vi "Main Monitor Loop.vi"(5 "tdms file out":refnum<k34>, 7 "Message Queue":refnum<queue>, 8 "error in (no error)":errorcluster, 10 "DATA ARRAY":dbl[][](array[numeric]), 11 "main ref":T1) -> (0 "error out":errorcluster, 2 "DATA ARRAY OUT":dbl[][](array[numeric]))   [LabVIEW 2025]
uses:
  v06/controls/LAB-IQ UI Data.ctl
  Traction Loop/Traction Receipe Enum.ctl
  support/Message Queue/Message Cluster.ctl
  Temperature/Temperature enum.ctl
  <vilib>/Utility/error.llb/Trim Whitespace One-Sided.vi
  support/Message Queue/Enqueue Message (Single).vi
  support/Message Queue/LAB-IQ Message Queue.lvlib
panel:
  out "error out 4":errorcluster
  out "ELAPSED INDICATION":bool
  out "error out 3":errorcluster
  out "output array":dbl[][](array[numeric])
  out "error out 2":errorcluster
  in  "Checkbox":bool
  out "Time elapsed":bool
  out "Test Stop Temp":bool
  out "DepthZ":dbl
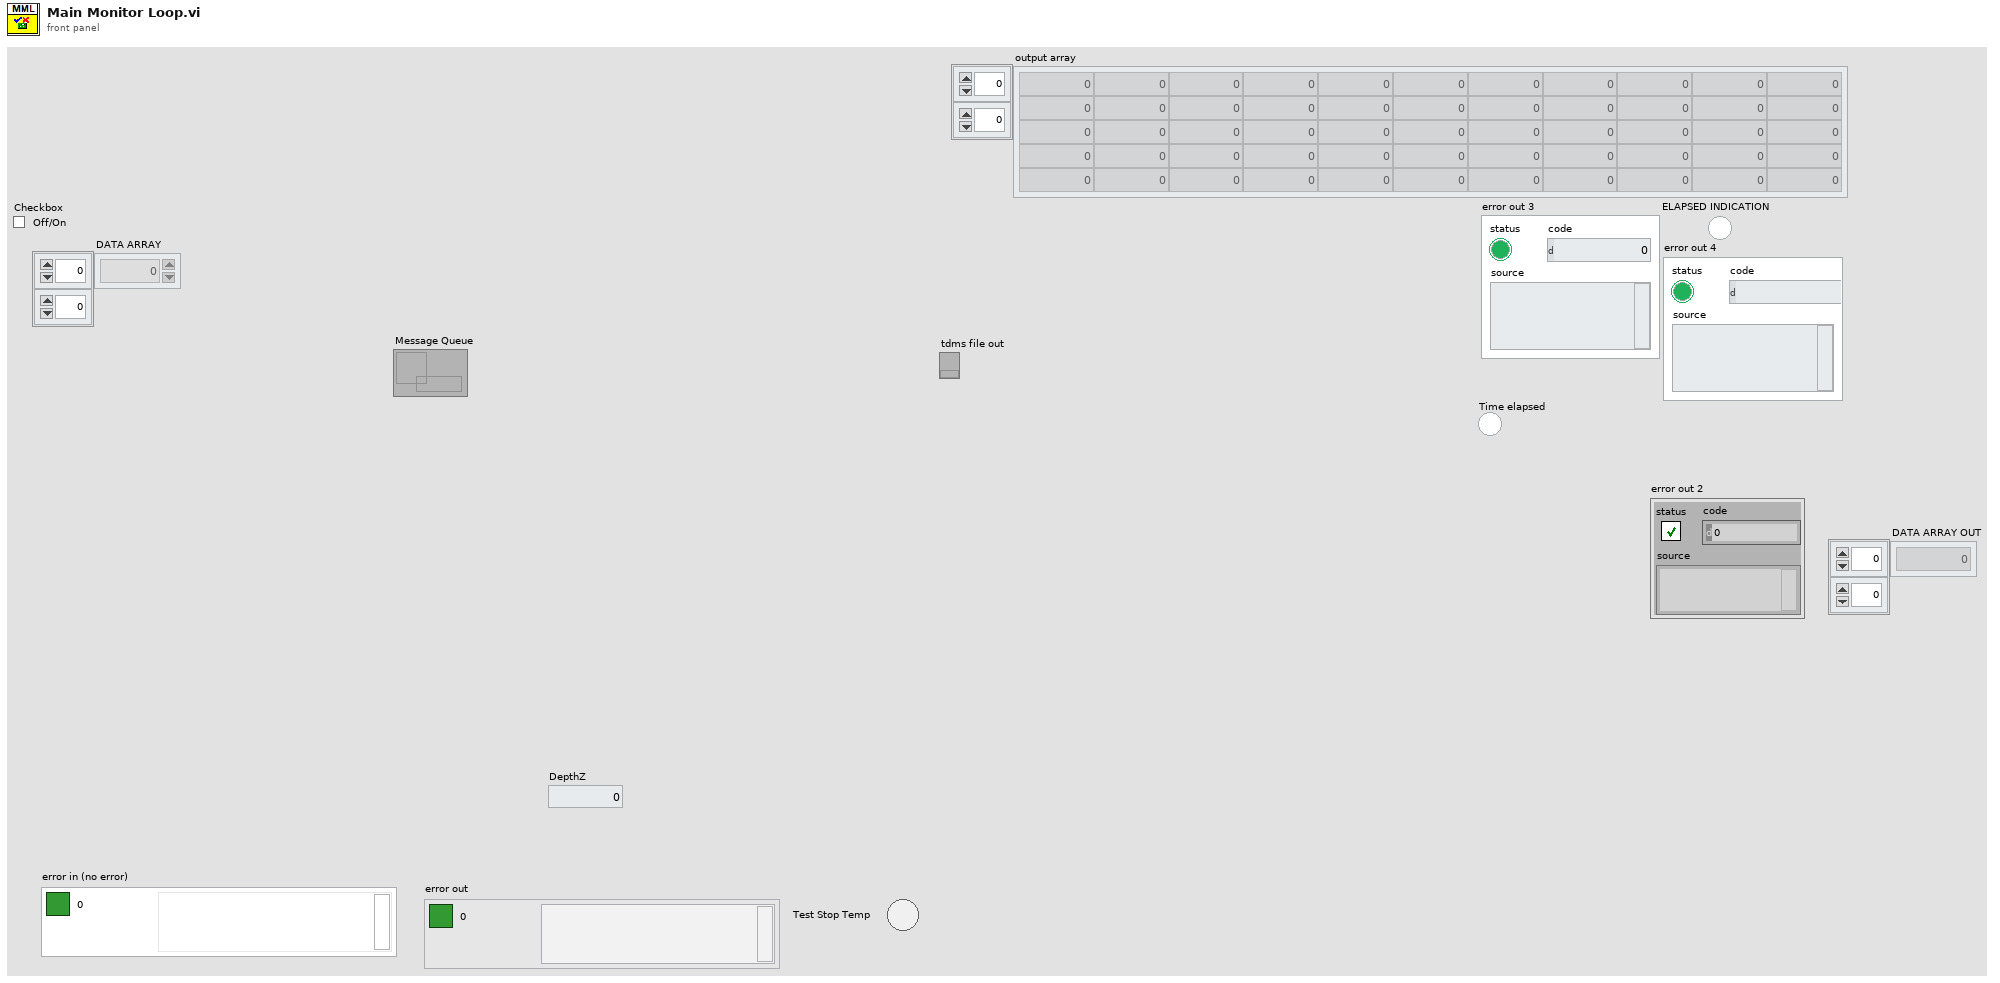
[diagram p1: front panel]
types:
  T1 = typedef "LAB-IQ UI Data.ctl" = cluster{"Main Home Screen":cluster{"GUI":refnum<vi>, "Platform Settings":refnum<vi>, "Configure":refnum<vi>, "Home":refnum<vi>, "EXIT":refnum<vi>, "service 2":refnum<vi>, "MainPage":refnum<vi>, "Analysis":refnum<vi>}, "Platform Settings":cluster{"mm/s  Surge":refnum<vi>, "Drive Error":refnum<vi>, "Disable Axis Jog Soft Limits":refnum<vi>, "mm/s  Sway":refnum<vi>, "Sway and Surge COM Status":refnum<vi>, "Heave COM Status":refnum<vi>, "Enable Platform":refnum<vi>, "Surge Forward Main":refnum<vi>, "Sway Right Main":refnum<vi>, "Sway Left Main":refnum<vi>, "Heave Down Main":refnum<vi>, "Heave Up main":refnum<vi>, "mm/s Heave":refnum<vi>, "mm/sec":refnum<vi>, "mm":refnum<vi>, "Surge Backward Main":refnum<vi>}, "Analysis Screen":cluster{"Analysis Home":refnum<vi>, "Surface Analysis":refnum<vi>, "Imaging":refnum<vi>, "Image Analysis":refnum<vi>, "Post Analysis":refnum<vi>}, "Config Screen":cluster{"Select Load Head":refnum<vi>, "Notes :":refnum<vi>, "FILE":refnum<vi>, "Sample ID :":refnum<vi>, "Operator ID :":refnum<vi>, "Operator Name :":refnum<vi>, "Auto":refnum<vi>}, "Motion Module":cluster{"zNL":refnum<vi>, "NL disp":refnum<vi>, "Rotary Tab":refnum<vi>, "Motion Direction:  3":refnum<vi>, "E.Velocity 2":refnum<vi>, "e.v/ssr 2":refnum<vi>, "Enter Fixed E.Velocity 2":refnum<vi>, "Enter Final SRR 2":refnum<vi>, "Enter initial SRR 2":refnum<vi>, "Enter Fixed SRR 2":refnum<vi>, "Enter the Final E.Velocity (m/s) 2":refnum<vi>, "Enter initial E.Velocity (m/s) 2":refnum<vi>, "Final Speed (RPM) 3":refnum<vi>, "Initial Speed (RPM) 2":refnum<vi>, "Enter the Final Velocity (m/s) 3":refnum<vi>, "Enter initial Velocity (m/s)  3":refnum<vi>, "Ramp Up 2":refnum<vi>, "TEST SELECTION":refnum<vi>, "SPEED SELECTION : ":refnum<vi>, "Angular Oscillation Set":refnum<vi>, "Traction":refnum<vi>, "Step Speed":refnum<vi>, "StepTable For Load-Speed":refnum<vi>, "StepTable For Speed":refnum<vi>, "Surge Forward MM":refnum<vi>, "Surge Backward MM":refnum<vi>, "M3 Image":refnum<vi>, "String 39":refnum<vi>, "Sway Left MM":refnum<vi>, "Sway Right MM":refnum<vi>, "Disable Axis Jog Soft Limits":refnum<vi>, "mm":refnum<vi>, "Heave Down MM":refnum<vi>, "Heave Up MM":refnum<vi>, "Wear Track Diameter (mm)":refnum<vi>, "Set WTD":refnum<vi>, "HomeScratch":refnum<vi>, "HomeRot":refnum<vi>, "PlaceModule":refnum<vi>, "Enter the Angle (Deg)":refnum<vi>, "Enter the Frequency (Hz)":refnum<vi>, "Motion Mode:":refnum<vi>, "LR Sway":refnum<vi>, "Rot Hor":refnum<vi>, "Scratch":refnum<vi>, "LR Cam":refnum<vi>, "MMBack":refnum<vi>, "MMNext":refnum<vi>, "Rot Ver":refnum<vi>, "Rotary Module Selection":refnum<vi>, "calculate rotary":refnum<vi>, "SPEED SELECTION : rotary":refnum<vi>, "Import 2":refnum<vi>, "Save 2":refnum<vi>, "File Path :  2":refnum<vi>, "String 45":refnum<vi>, "StepTable For Speed 3":refnum<vi>, "Enter the Speed(mm/sec)":refnum<vi>, "Enter the Speed(RPM)":refnum<vi>, "Enter Scratch Speed (mm/s):":refnum<vi>, "SwaySpeed Set":refnum<vi>, "Scartch Offset":refnum<vi>, "Motion type:":refnum<vi>, "HomeScratch 2":refnum<vi>, "Enter Scratch length (mm):":refnum<vi>, "Wear Track Diameter":refnum<vi>, "Rotary Speed Exced":refnum<vi>, "Scratch Mode":refnum<vi>, "No of Scratch":refnum<vi>}, "Environmental control":cluster{"Humidity  Status  3":refnum<vi>, "Low Temp  Status  2":refnum<vi>, "TK4 status 2":refnum<vi>, "Stage Temperature":refnum<vi>, "Sample Temperature":refnum<vi>, "Humidity (Amb)":refnum<vi>, "Clear List":refnum<vi>, "Add to list":refnum<vi>, "Wear":refnum<vi>, "Vibration":refnum<vi>, "Humidity (Chamber)":refnum<vi>, "Temperature (Chamber)":refnum<vi>, "ECR ":refnum<vi>, "Temperature (Amb)":refnum<vi>, "Microphone":refnum<vi>, "Acoustic Emission 3":refnum<vi>, "SNext":refnum<vi>, "APBack":refnum<vi>, "Enter the Temperature (°C):":refnum<vi>, "Enter the Stage \nTemperature (°C):":refnum<vi>, "Enter the Humidity (%Rh):":refnum<vi>, "Low Temp":refnum<vi>, "High Temp":refnum<vi>, "Humidity":refnum<vi>, "Sensors Picked":refnum<vi>}, "About Screen":cluster{"Password":refnum<vi>, "Home Service":refnum<vi>, "Advanced Setting":refnum<vi>, "About Tab":refnum<vi>, "ECR Port:":refnum<vi>, "Ramp Port:":refnum<vi>, "Installation/Replacement completed":refnum<vi>, "Loahead":refnum<vi>, "Heave and Surge COM Port:":refnum<vi>, "Sway COM Port:":refnum<vi>, "Temp Modbus:":refnum<vi>, "Humidity Port:":refnum<vi>, "Edit Gain Constants":refnum<vi>, "Save Gain Constants":refnum<vi>}, "Main Screen":cluster{"Main Screen Tab":refnum<vi>, "Angle and Frequency":refnum<vi>, "Stroke (mm)":refnum<vi>, "Angle (Deg)":refnum<vi>, "Main Speed Tab":refnum<vi>, "MTM MOTOR DISPLAY":refnum<vi>, "Disc Speed (m/sec)":refnum<vi>, "Ball Speed (m/sec)":refnum<vi>, "Disc Speed (RPM)":refnum<vi>, "Ball Speed (RPM)":refnum<vi>, "SPEED TAB":refnum<vi>, "Speed (m/sec)":refnum<vi>, "Set Speed (m/sec)":refnum<vi>, "Speed (RPM)":refnum<vi>, "Set Speed":refnum<vi>, "Time Tab":refnum<vi>, "Time ( HH:MM:SS ) 2":refnum<vi>, "Test Duration":refnum<vi>, "Test Duration 4":refnum<vi>, "TEST CYCLE":refnum<vi>, "TOTAL CYCLES":refnum<vi>, "Set Load (N)":refnum<vi>, "Temp Tabs":refnum<vi>, "Heater":refnum<vi>, "TK4 status":refnum<vi>, "ChamberTemp":refnum<vi>, "SetTmp":refnum<vi>, "Controller  Status":refnum<vi>, "ChamberTemp 2":refnum<vi>, "SetTmp 2":refnum<vi>, "Controller  Status 2":refnum<vi>, "ChamberTemp 3":refnum<vi>, "SetTmp 3":refnum<vi>, "Cooling":refnum<vi>, "Load Communication":refnum<vi>, "Ambient \nTemperature":refnum<vi>, "HumCOMStatus":refnum<vi>, "Ambient\n Humidity":refnum<vi>, "Freq (Hz)":refnum<vi>, "Load En":refnum<vi>, "NLt":refnum<vi>, "zNL 2":refnum<vi>, "Humidity On":refnum<vi>, "humidity disp":refnum<vi>, "Set Humidity":refnum<vi>, "NL disp 2":refnum<vi>, "Humidity On 2":refnum<vi>, "humidity disp 2":refnum<vi>, "Set Humidity 2":refnum<vi>, "NL disp 3":refnum<vi>, "AppLoadSeq scratch":refnum<vi>, "Stop Scratch":refnum<vi>, "ClrLog":refnum<vi>, "Trip Log":refnum<vi>, "STOP":refnum<vi>, "Start Test":refnum<vi>, "Test status":refnum<vi>, "AR Led":refnum<vi>, "Data":refnum<vi>, "Health":refnum<vi>, "Sway COM Status":refnum<vi>, "Heave COM Status":refnum<vi>, "Grp Tab":refnum<vi>, "Sub Graph":refnum<vi>, "SD (mm)":refnum<vi>, "Siliding distance Reset Graph":refnum<vi>, "SDGp":refnum<vi>, "Humidity Reset Graph":refnum<vi>, "HumrGp":refnum<vi>, "Acoustic Emission (mV)":refnum<vi>, "Aqucostic Reset Graph":refnum<vi>, "gACQUOS":refnum<vi>, "ECR RESET":refnum<vi>, "ECR":refnum<vi>, "Temperature Reset":refnum<vi>, "Acoustic Emission (mV) 2":refnum<vi>, "Aqucostic Reset Graph 2":refnum<vi>, "gACQUOS 2":refnum<vi>, "ECR RESET 2":refnum<vi>, "ECR 2":refnum<vi>, "Temperature Reset 2":refnum<vi>, "Temperature (deg c)":refnum<vi>, "Speed Reset Graph":refnum<vi>, "Speed Tab":refnum<vi>, "MTM DISC  SPEED":refnum<vi>, "MTM BALL SPEED":refnum<vi>, "speed mm/sec":refnum<vi>, "Hymidity":refnum<vi>, "Humidity Disable trip":refnum<vi>, "CoF Trip  2":refnum<vi>, "Depth Trip":refnum<vi>, "Weart Deapth":refnum<vi>, "Depth Reset Graph":refnum<vi>, "Weart":refnum<vi>, "Depthz":refnum<vi>, "Depth (µm)":refnum<vi>, "WearGp":refnum<vi>, "NL Trip 2":refnum<vi>, "Load pid":refnum<vi>, "Load Disable Trip":refnum<vi>, "Load Reset Graph":refnum<vi>, "NL Display 4":refnum<vi>, "Main Chart 3":refnum<vi>, "BACK":refnum<vi>, "Depth Trip 2":refnum<vi>, "COF TRIP ":refnum<vi>, "Friction Force (N)":refnum<vi>, "FF Reset Graph":refnum<vi>, "FF Disable Trip":refnum<vi>, "FF TRIP":refnum<vi>, "COF Disable Trip":refnum<vi>, "COF Reset Graph":refnum<vi>, "Start Test Temp":refnum<vi>, "zFF":refnum<vi>, "Friction Force (N) Graph":refnum<vi>, "Coefficient of Friction":refnum<vi>, "Scratch Start Test":refnum<vi>, "FF Tab":refnum<vi>, "Cyclic Friction Force (N)":refnum<vi>, "CZ FF":refnum<vi>, "Cyclic Friction Force (N) Graph":refnum<vi>, "Cyclic Coefficient of Friction":refnum<vi>, "Cyclic FF TRIP":refnum<vi>, "Cyclic FF Disable Trip":refnum<vi>, "cyclic COF Disable Trip":refnum<vi>, "cyclic COF TRIP":refnum<vi>, "cyclic COF Reset Graph":refnum<vi>, "Cyclic FF Reset Graph":refnum<vi>, "Test Trip":refnum<vi>, "Multi Scratch Pass":refnum<vi>, "Scratch Start Recording":refnum<vi>, "Coefficient of Friction 2":refnum<vi>, "Acoustic Emission":refnum<vi>, "Friction Force (N) 2":refnum<vi>, "Depth (Microns)":refnum<vi>, "Normal Load ( N )":refnum<vi>}, "Loading":cluster{"Indentation":refnum<vi>, "Reference Sample":refnum<vi>, "Load Cell Communication Slide":refnum<vi>, "com 3":refnum<vi>, "com":refnum<vi>, "DecaForce COM Status":refnum<vi>, "Update":refnum<vi>, "Clear 3":refnum<vi>, "seq":refnum<vi>, "Stribeck table":refnum<vi>, "Stribeck Table  For loading":refnum<vi>, "Loading Mode":refnum<vi>, "Enter the Final Load (N)":refnum<vi>, "Enter the CoF Trip":refnum<vi>, "Enter the Friction Force Trip":refnum<vi>, "Enter the Normal load Trip":refnum<vi>, "Enter the Load  (N)":refnum<vi>, "KiloForce":refnum<vi>, "DecaForce ":refnum<vi>, "MicroForce":refnum<vi>, "LHBack":refnum<vi>, "LHNext":refnum<vi>, "Enter the Loading Rate (N/min)":refnum<vi>, "Message":refnum<vi>, "Warning 2":refnum<vi>, "SSP 0.75":refnum<vi>, "SSP 0.5":refnum<vi>, "SSP 0.3":refnum<vi>, "Warning":refnum<vi>, "gui GIF":refnum<vi>, "Communication is established":refnum<vi>, "AppLoad 4":refnum<vi>, "Multipoint":refnum<vi>, "Load Selection":refnum<vi>}, "PID":cluster{"Ramp":refnum<vi>, "Vertical load (N)":refnum<vi>, "apply load":refnum<vi>, "apply load 2":refnum<vi>, "Enter ByPass Load":refnum<vi>, "Bypass Load":refnum<vi>, "gFF Rot":refnum<vi>}, "Config Parameters":cluster{"Tab Control 3":refnum<vi>, "Tab Control 19":refnum<vi>, "SAMPLES":refnum<vi>, "Re-initilaize":refnum<vi>, "Filter ON/OFF":refnum<vi>, "TracHomeSurgeOffsetCounts 10MM":refnum<vi>, "TracHomeSwayOffsetCounts 10MM":refnum<vi>, "Acoustic Emission:":refnum<vi>, "Apply Filter (FF)":refnum<vi>, "Filter% 2":refnum<vi>, "Apply Filter (Load)":refnum<vi>, "Filter% ":refnum<vi>, "Sway distance (mm)":refnum<vi>, "Surge distance (mm)":refnum<vi>, "DataSavingLoopDelay(ms)":refnum<vi>, "SAVE 2":refnum<vi>, "Enter Distance":refnum<vi>, "Sway Counts:":refnum<vi>, "Distance (mm): 3":refnum<vi>, "Surge Counts:":refnum<vi>, "Distance (mm): 2":refnum<vi>, "Distance (mm):":refnum<vi>, "Heave Counts:":refnum<vi>, "LRMHomeSurgeOffsetCounts":refnum<vi>, "LRMHomeSwayOffsetCounts":refnum<vi>, "TracHomeSurgeOffsetCounts 20MM":refnum<vi>, "TracHomeSwayOffsetCounts 20MM":refnum<vi>, "RotHomeSwayOffsetCounts":refnum<vi>, "RotHomeSurgeOffsetCounts":refnum<vi>, "Heave distance":refnum<vi>, "Zmm":refnum<vi>, "Heave Pulses/mm":refnum<vi>, "Surge Pulses/mm":refnum<vi>, "Sway Pulses/mm":refnum<vi>, "Heave Pitch":refnum<vi>, "Surge Pitch":refnum<vi>, "Sway Pitch":refnum<vi>, "Heave PPR":refnum<vi>, "Surge PPR":refnum<vi>, "Sway PPR":refnum<vi>, "Tab Control 5":refnum<vi>, "Tab Control 14":refnum<vi>, "Tab Control 26":refnum<vi>, "AE":refnum<vi>, "Heave Loop Delay":refnum<vi>, "Heave PID Speed":refnum<vi>, "Surge Jog Speed":refnum<vi>, "Heave Jog Speed":refnum<vi>, "Sway Loop Delay":refnum<vi>, "Sway PID Speed":refnum<vi>, "Sway Jog Speed":refnum<vi>, "DEPTH TRIP VALUE":refnum<vi>, "LOAD TRIP VALUE":refnum<vi>, "DEPTH TRIP   ENABLE":refnum<vi>, "LOAD TRIP  ENABLE":refnum<vi>, "CYCLIC FF TRIP VALUE":refnum<vi>, "FF TRIP VALUE":refnum<vi>, "CYCLIC CoF TRIP VALUE":refnum<vi>, "COF TRIP VALUE":refnum<vi>, "CYCLIC COF TRIP  ENABLE":refnum<vi>, "CYCLIC FF TRIP  ENABLE":refnum<vi>, "FF TRIP  ENABLE":refnum<vi>, "COF TRIP  ENABLE":refnum<vi>, "JOG TRIP LOAD VALUE (N)":refnum<vi>, "Rotary Vertical":refnum<vi>, "Traction":refnum<vi>, "Scratch":refnum<vi>, "LRM CAM":refnum<vi>, "Sway LRM":refnum<vi>, "Rotary Horizontal":refnum<vi>, "SURGE SPEED":refnum<vi>, "SURGE BACKWARD COUNT":refnum<vi>, "SURGE FORWARD COUNT":refnum<vi>, "Start Button":refnum<vi>}, "Loading Com Port":cluster{"ClearAll":refnum<vi>, "Mz(Nm)":refnum<vi>, "My(Nm)":refnum<vi>, "Mx(Nm)":refnum<vi>, "Save Dwell":refnum<vi>, "Acq Delay (ms)":refnum<vi>, "Burst Delay (ms)":refnum<vi>, "model":refnum<vi>, "SN":refnum<vi>, "FFx(N)":refnum<vi>, "Sensor IP":refnum<vi>, "Port":refnum<vi>, "FFy(N)":refnum<vi>, "Load(N)":refnum<vi>, "delete Handle":refnum<vi>, "Create Handle":refnum<vi>, "ft_data":refnum<vi>, "ft_range":refnum<vi>, "ft_data 2":refnum<vi>, "stop 6":refnum<vi>, "running_flag":refnum<vi>, "ft_udp_handle":refnum<vi>, "get-data-return":refnum<vi>, "get-range-return":refnum<vi>, "zero-return":refnum<vi>, "filter-return":refnum<vi>, "initial-return":refnum<vi>, "deleteHandle-result":refnum<vi>, "Load Cell Temp":refnum<vi>, "Load Cell":refnum<vi>, "ZeroAll":refnum<vi>, "FORCE (N)":refnum<vi>, "TORQUE (N-m)":refnum<vi>, "Load Cell Link":refnum<vi>}, "Heave AND Surge":cluster{"SURGE POSE":refnum<vi>, "error out Read":refnum<vi>, "HEAVE POSE":refnum<vi>, "State":refnum<vi>, "Homed":refnum<vi>, "Sequence ID":refnum<vi>, "error out Write":refnum<vi>, "faultCode":refnum<vi>, "Ack ID":refnum<vi>, "SPEED":refnum<vi>, "Distance":refnum<vi>, "Mode Command":refnum<vi>, "Heave and Surge Read":refnum<vi>, "Read Heave Temp":refnum<vi>, "Spare 15":refnum<vi>, "Spare 14":refnum<vi>, "Spare 13":refnum<vi>, "Spare 12":refnum<vi>, "Spare 11":refnum<vi>, "Spare 10":refnum<vi>, "Spare 9":refnum<vi>, "Spare 8":refnum<vi>, "Spare 7":refnum<vi>, "Spare 4":refnum<vi>, "Spare 3":refnum<vi>, "Spare 2":refnum<vi>, "Humidity":refnum<vi>, "Temp":refnum<vi>, "Node Id":refnum<vi>, "Spare 1":refnum<vi>, "SPARE 4":refnum<vi>, "SPARE 3":refnum<vi>, "SPARE 2":refnum<vi>, "SPARE 1":refnum<vi>, "fwMajor":refnum<vi>, "fwMinor":refnum<vi>, "Manual Write":refnum<vi>, "Heave and Surge Write":refnum<vi>, "SPARE 5":refnum<vi>, "Reserved ":refnum<vi>, "SPARE 8":refnum<vi>, "SPARE 6":refnum<vi>, "SPARE 7":refnum<vi>, "SPARE 17":refnum<vi>, "SPARE 16":refnum<vi>, "SPARE 15":refnum<vi>, "SPARE 14":refnum<vi>, "SPARE 13":refnum<vi>, "SPARE 12":refnum<vi>, "SPARE 11":refnum<vi>, "SPARE 10":refnum<vi>, "SPARE 9":refnum<vi>, "System UPTIME":refnum<vi>, "Missed Packets":refnum<vi>, "faultCode Surge Right":refnum<vi>, "faultCode Surge Left":refnum<vi>, "faultCode Heave":refnum<vi>, "UPLINK HEAVE":refnum<vi>, "DOWNLINK HEAVE":refnum<vi>}, "New PID LOGIC":cluster{"Fine Tune Zone":refnum<vi>, "PID SDelay":refnum<vi>, "Max_pos_limit":refnum<vi>, "Min_pos_limit":refnum<vi>, "i_limit":refnum<vi>, "pct_scale":refnum<vi>, "Deadband":refnum<vi>, "Kd":refnum<vi>, "Ki":refnum<vi>, "Kp":refnum<vi>, "Current Position":refnum<vi>, "Set Load":refnum<vi>, "Current Load":refnum<vi>, "Pulse delta":refnum<vi>, "Init Step":refnum<vi>, "Max Step Linit":refnum<vi>, "min_deadband_floor":refnum<vi>, "dynamic_spindle_noise_scalar":refnum<vi>, "min_finetune_floor":refnum<vi>, "filter_alpha":refnum<vi>, "PID":refnum<vi>}, "SWAY ":cluster{"fwMajor":refnum<vi>, "Homed":refnum<vi>, "Rotary POSE":refnum<vi>, "State":refnum<vi>, "SWAY POSE":refnum<vi>, "Ack ID":refnum<vi>, "faultCode":refnum<vi>, "Node Id":refnum<vi>, "fwMinor":refnum<vi>, "Spare 6":refnum<vi>, "Spare 5":refnum<vi>, "Spare 4":refnum<vi>, "Spare 3":refnum<vi>, "Spare 2":refnum<vi>, "Spare 1":refnum<vi>, "Spare 7":refnum<vi>, "SPARE  5":refnum<vi>, "error out Write  SWAY ":refnum<vi>, "error out Read SWAY ":refnum<vi>, "Manual Write SWAY ":refnum<vi>, "SWAY WRITE":refnum<vi>, "SPARE  4":refnum<vi>, "SPARE  3":refnum<vi>, "SPARE 2":refnum<vi>, "SPARE 1":refnum<vi>, "Spare 15":refnum<vi>, "Spare 14":refnum<vi>, "Spare 13":refnum<vi>, "Spare 12":refnum<vi>, "Spare 11":refnum<vi>, "Spare 9":refnum<vi>, "Spare 8":refnum<vi>, "SPEED":refnum<vi>, "Distance":refnum<vi>, "Mode Command":refnum<vi>, "Sequence ID":refnum<vi>, "SWAY READ":refnum<vi>, "Spare 10":refnum<vi>, "Read SWAY Temp":refnum<vi>, "faultCode Sway ":refnum<vi>, "Missed Packets":refnum<vi>, "System UPTIME sway":refnum<vi>, "SPARE 6":refnum<vi>, "SPARE 7":refnum<vi>, "SPARE 9":refnum<vi>, "SPARE 11":refnum<vi>, "SPARE 10":refnum<vi>, "SPARE 8":refnum<vi>, "SPARE 13":refnum<vi>, "SPARE 12":refnum<vi>, "SPARE 17":refnum<vi>, "SPARE 16":refnum<vi>, "SPARE 15":refnum<vi>, "SPARE 14":refnum<vi>, "Reserved":refnum<vi>, "faultCode Rotary":refnum<vi>, "UPLINK SWAY":refnum<vi>, "DOWNLINK SWAY":refnum<vi>}, "Analysis Screen":cluster{"Analysis Home":refnum<vi>, "Refresh 2":refnum<vi>, "MEAN 4":refnum<vi>, "SD 4":refnum<vi>, "VARIANCE 4":refnum<vi>, "MEAN  3":refnum<vi>, "SD  3":refnum<vi>, "VARIANCE  3":refnum<vi>, "MEAN 2":refnum<vi>, "SD  2":refnum<vi>, "VARIANCE 2":refnum<vi>, "MEAN":refnum<vi>, "SD":refnum<vi>, "VARIANCE":refnum<vi>, "File 4 Discription":refnum<vi>, "OPEN 4":refnum<vi>, "File Name 4":refnum<vi>, "OPEN 3":refnum<vi>, "File 3 Discription":refnum<vi>, "File Name 3":refnum<vi>, "Y-AXIS":refnum<vi>, "X-AXIS":refnum<vi>, "XY Graph":refnum<vi>, "File Name 2":refnum<vi>, "File Name 1":refnum<vi>, "OPEN 2":refnum<vi>, "OPEN 1":refnum<vi>, "File 1 Discription ":refnum<vi>, "File 2 Discription":refnum<vi>, "Export":refnum<vi>, "File Format":refnum<vi>}, "Traction":cluster{"faultCode Traction 2":refnum<vi>, "faultCode Traction 1":refnum<vi>, "Missed Packets":refnum<vi>, "System UPTIME Traction":refnum<vi>, "SPARE 17":refnum<vi>, "SPARE 16":refnum<vi>, "SPARE 15":refnum<vi>, "SPARE 14":refnum<vi>, "SPARE 13":refnum<vi>, "SPARE 12":refnum<vi>, "SPARE 11":refnum<vi>, "SPARE 10":refnum<vi>, "SPARE 9":refnum<vi>, "SPARE 8":refnum<vi>, "SPARE 7":refnum<vi>, "SPARE 6":refnum<vi>, "Reserved":refnum<vi>, "SPARE  5":refnum<vi>, "Manual Write TRACTION":refnum<vi>, "TRACTION WRITE":refnum<vi>, "SPARE  4":refnum<vi>, "SPARE  3":refnum<vi>, "SPARE 2":refnum<vi>, "SPARE 1":refnum<vi>, "Spare 7":refnum<vi>, "Spare 6":refnum<vi>, "Spare 5":refnum<vi>, "Spare 4":refnum<vi>, "Spare 2":refnum<vi>, "Spare 1":refnum<vi>, "Node Id":refnum<vi>, "Read TRACTION Temp":refnum<vi>, "fwMinor":refnum<vi>, "fwMajor":refnum<vi>, "faultCode":refnum<vi>, "TRACTION POSE":refnum<vi>, "TRACTION POSE 2":refnum<vi>, "Homed":refnum<vi>, "State":refnum<vi>, "Ack ID":refnum<vi>, "SPEED":refnum<vi>, "Distance":refnum<vi>, "Mode Command":refnum<vi>, "Sequence ID":refnum<vi>, "error out Read TRACTION":refnum<vi>, "error out Write  TRACTION":refnum<vi>, "TRACTION READ":refnum<vi>, "Spare 3":refnum<vi>, "Downlink traction":refnum<vi>, "Uplink Traction":refnum<vi>}, "Traction reciepe":cluster{"SRR Sweep Range (%) Stribeck":refnum<vi>, "Traction Receipe":refnum<vi>, "Total Execution Time":refnum<vi>, "Total Steps":refnum<vi>, "Duration / Step (s)  Stribeck":refnum<vi>, "STRIBECK Fixed SRR List (%)":refnum<vi>, "Duration / Step (s) Traction":refnum<vi>, "SRR Sweep Range (%) traction":refnum<vi>, "Rolling Speed (mm/s)":refnum<vi>, "Temperature Stages (°C)":refnum<vi>, "Ball Load (N)":refnum<vi>, "Lubricant Name":refnum<vi>, "Profile File Name":refnum<vi>, "SET entrainment Velocity":refnum<vi>, "Test Array Size":refnum<vi>, "SRR INDEX [ STRIBECK]":refnum<vi>, "Stribeck Size":refnum<vi>, "SET SRR":refnum<vi>, "ELAPSED TIMER ":refnum<vi>, "BALL SET RPM":refnum<vi>, "DISC SET RPM":refnum<vi>, "SET LOAD":refnum<vi>, "TEMPERATURE READ":refnum<vi>, "SET TEMPERATURE":refnum<vi>, "Traction Size":refnum<vi>, "DISC SPEED (rpm)":refnum<vi>, "BALL SPEED (rpm)":refnum<vi>, "BALL WEAR TRACK":refnum<vi>, "DISC WEARTRACK":refnum<vi>, "SRR INDEX [ TRACTION]":refnum<vi>, "Start Index Type":refnum<vi>, "Enum - Menu":refnum<vi>, "Ball (mm/sec)":refnum<vi>, "Disc (mm/sec)":refnum<vi>, "Traction Receipe Update Details":refnum<vi>}, "Traction Control":cluster{"HomeTraction":refnum<vi>, "Demo Mode Display":refnum<vi>, "Traction Message":refnum<vi>, "Traction Step Update Details":refnum<vi>, "Main Tab sequence for selection":refnum<vi>, "Ramp Tab":refnum<vi>, "e.v/ssr":refnum<vi>, "Enter Fixed E.Velocity":refnum<vi>, "Enter Final SRR":refnum<vi>, "Enter initial SRR":refnum<vi>, "Enter Fixed SRR":refnum<vi>, "Enter the Final E.Velocity (m/s)":refnum<vi>, "Enter initial E.Velocity (m/s)":refnum<vi>, "Ball WTD":refnum<vi>, "E.Velocity":refnum<vi>, "Enter the Final Velocity (m/s)":refnum<vi>, "Enter initial Velocity (m/s)":refnum<vi>, "Ramp Up   Disc":refnum<vi>, "Initial DiscSpeed (RPM)":refnum<vi>, "Final Speed (RPM) Ball":refnum<vi>, "Final Speed (RPM)":refnum<vi>, "Initial Speed (RPM) Ball":refnum<vi>, "Enter the Final Velocity (m/s) Ball":refnum<vi>, "Enter initial Velocity (m/s) Ball":refnum<vi>, "Ramp Up":refnum<vi>, "ExceedBallSpeed step":refnum<vi>, "ExceedDiscSpeed":refnum<vi>, "BallSpeed Exceed Indication":refnum<vi>, "Apply":refnum<vi>, "SPEED SELECTION : MTM":refnum<vi>, "SPEED SELECTION : MTM 2":refnum<vi>, "TEST SELECTION (MTM)":refnum<vi>, "MTM Test Selection":refnum<vi>, "File Path Tab":refnum<vi>, "File Path String":refnum<vi>, "Save":refnum<vi>, "Save  2":refnum<vi>, "Import ":refnum<vi>, "File Path :":refnum<vi>, "Step Sequence Indication Tab":refnum<vi>, "Step Sequence Indication":refnum<vi>, "Calculate Step":refnum<vi>, "StepTable":refnum<vi>, "ExceedDiscSpeed  Cinstant Speed":refnum<vi>, "ExceedBallSpeed Constant":refnum<vi>, "TEST SELECTION (MTM) 2":refnum<vi>, "SPEED SELECTION : MTM 3":refnum<vi>, "MTM Test Selection 2":refnum<vi>, "Enter the Speed (m/sec): ":refnum<vi>, "Enter the Speed (m/sec):  2":refnum<vi>, "Enter the Speed (RPM):":refnum<vi>, "Lower Spped ":refnum<vi>, "Upper":refnum<vi>, "Enter the Speed (RPM):Ball":refnum<vi>, "Disc Motion Direction: ":refnum<vi>, "Ball Motion Direction :":refnum<vi>, "Motion Mode: ":refnum<vi>, "Wear Track Diameter (mm) ":refnum<vi>, "Disc Speed Indicator":refnum<vi>, "ExceedBallSpeed":refnum<vi>}, "Acquostic":cluster{"Last Config Rejected ":refnum<vi>, "rx command count":refnum<vi>, "Current Filter Id":refnum<vi>, "Isolated Gain":refnum<vi>, "DAQ Status":refnum<vi>, "error out":refnum<vi>, "error in (no error)":refnum<vi>, "Uplink Packet":refnum<vi>, "data out":refnum<vi>, "Downlink Packet":refnum<vi>, "Gains":refnum<vi>, "Manual Write Acquostic":refnum<vi>, "Acoustic Graphs":refnum<vi>}, "ABOUT":cluster{"version":refnum<vi>, "Operating System":refnum<vi>, "Version":refnum<vi>, "Workorder":refnum<vi>, "Runtime":refnum<vi>, "Instrument Serial":refnum<vi>, "Firmware Version":refnum<vi>, "Info":refnum<vi>}, "Temperature Port":cluster{"Temperature":refnum<vi>, "error out Temperature":refnum<vi>, "READ TEMPERATURE":refnum<vi>}}
  T2 = typedef "Temperature enum.ctl" = enum16{"Init", "read", "write", "close", "error_init"}
  T3 = cluster{"Ack ID":u16, "State":u8, "Homed":u8, "HEAVE POSE":sgl, "SURGE POSE":sgl, "faultCode":u16, "fwMajor":u8, "fwMinor":u8, "Node Id":u8, "Spare 1":u8, "Spare 2":u8, "Spare 3":u8, "Spare 4":u8, "Spare 5":u8, "Spare 6":u8, "Spare 7":u8, "System UPTIME":sgl, "Missed Packets":sgl, "faultCode Heave":u16, "faultCode Surge Left":u16, "faultCode Surge Right":u16}
  T4 = cluster{"Sequence ID":u32, "Timestamp":u32, "System Status":u32, "Peak Amplitude":sgl, "Amplitude dB_AE":sgl, "AE Ring-Down Counts":u32, "Signal Energy":sgl, "Spare 1":u32}
  T5 = cluster{"Ack ID ":u16, "State":u8, "Homed":u8, "SWAY POSE ":sgl, "Rotary POSE ":sgl, "faultCode":u16, "fwMajor":u8, "fwMinor":u8, "Node Id":u8, "Spare 1":u8, "Spare 2":u8, "Spare 3":u8, "Spare 4":u8, "Spare 5":u8, "Spare 6":u8, "Spare 7":u8, "System UPTIME ":sgl, "Missed Packets ":sgl, "faultCode Sway":u16, "faultCode Rotary":u16}
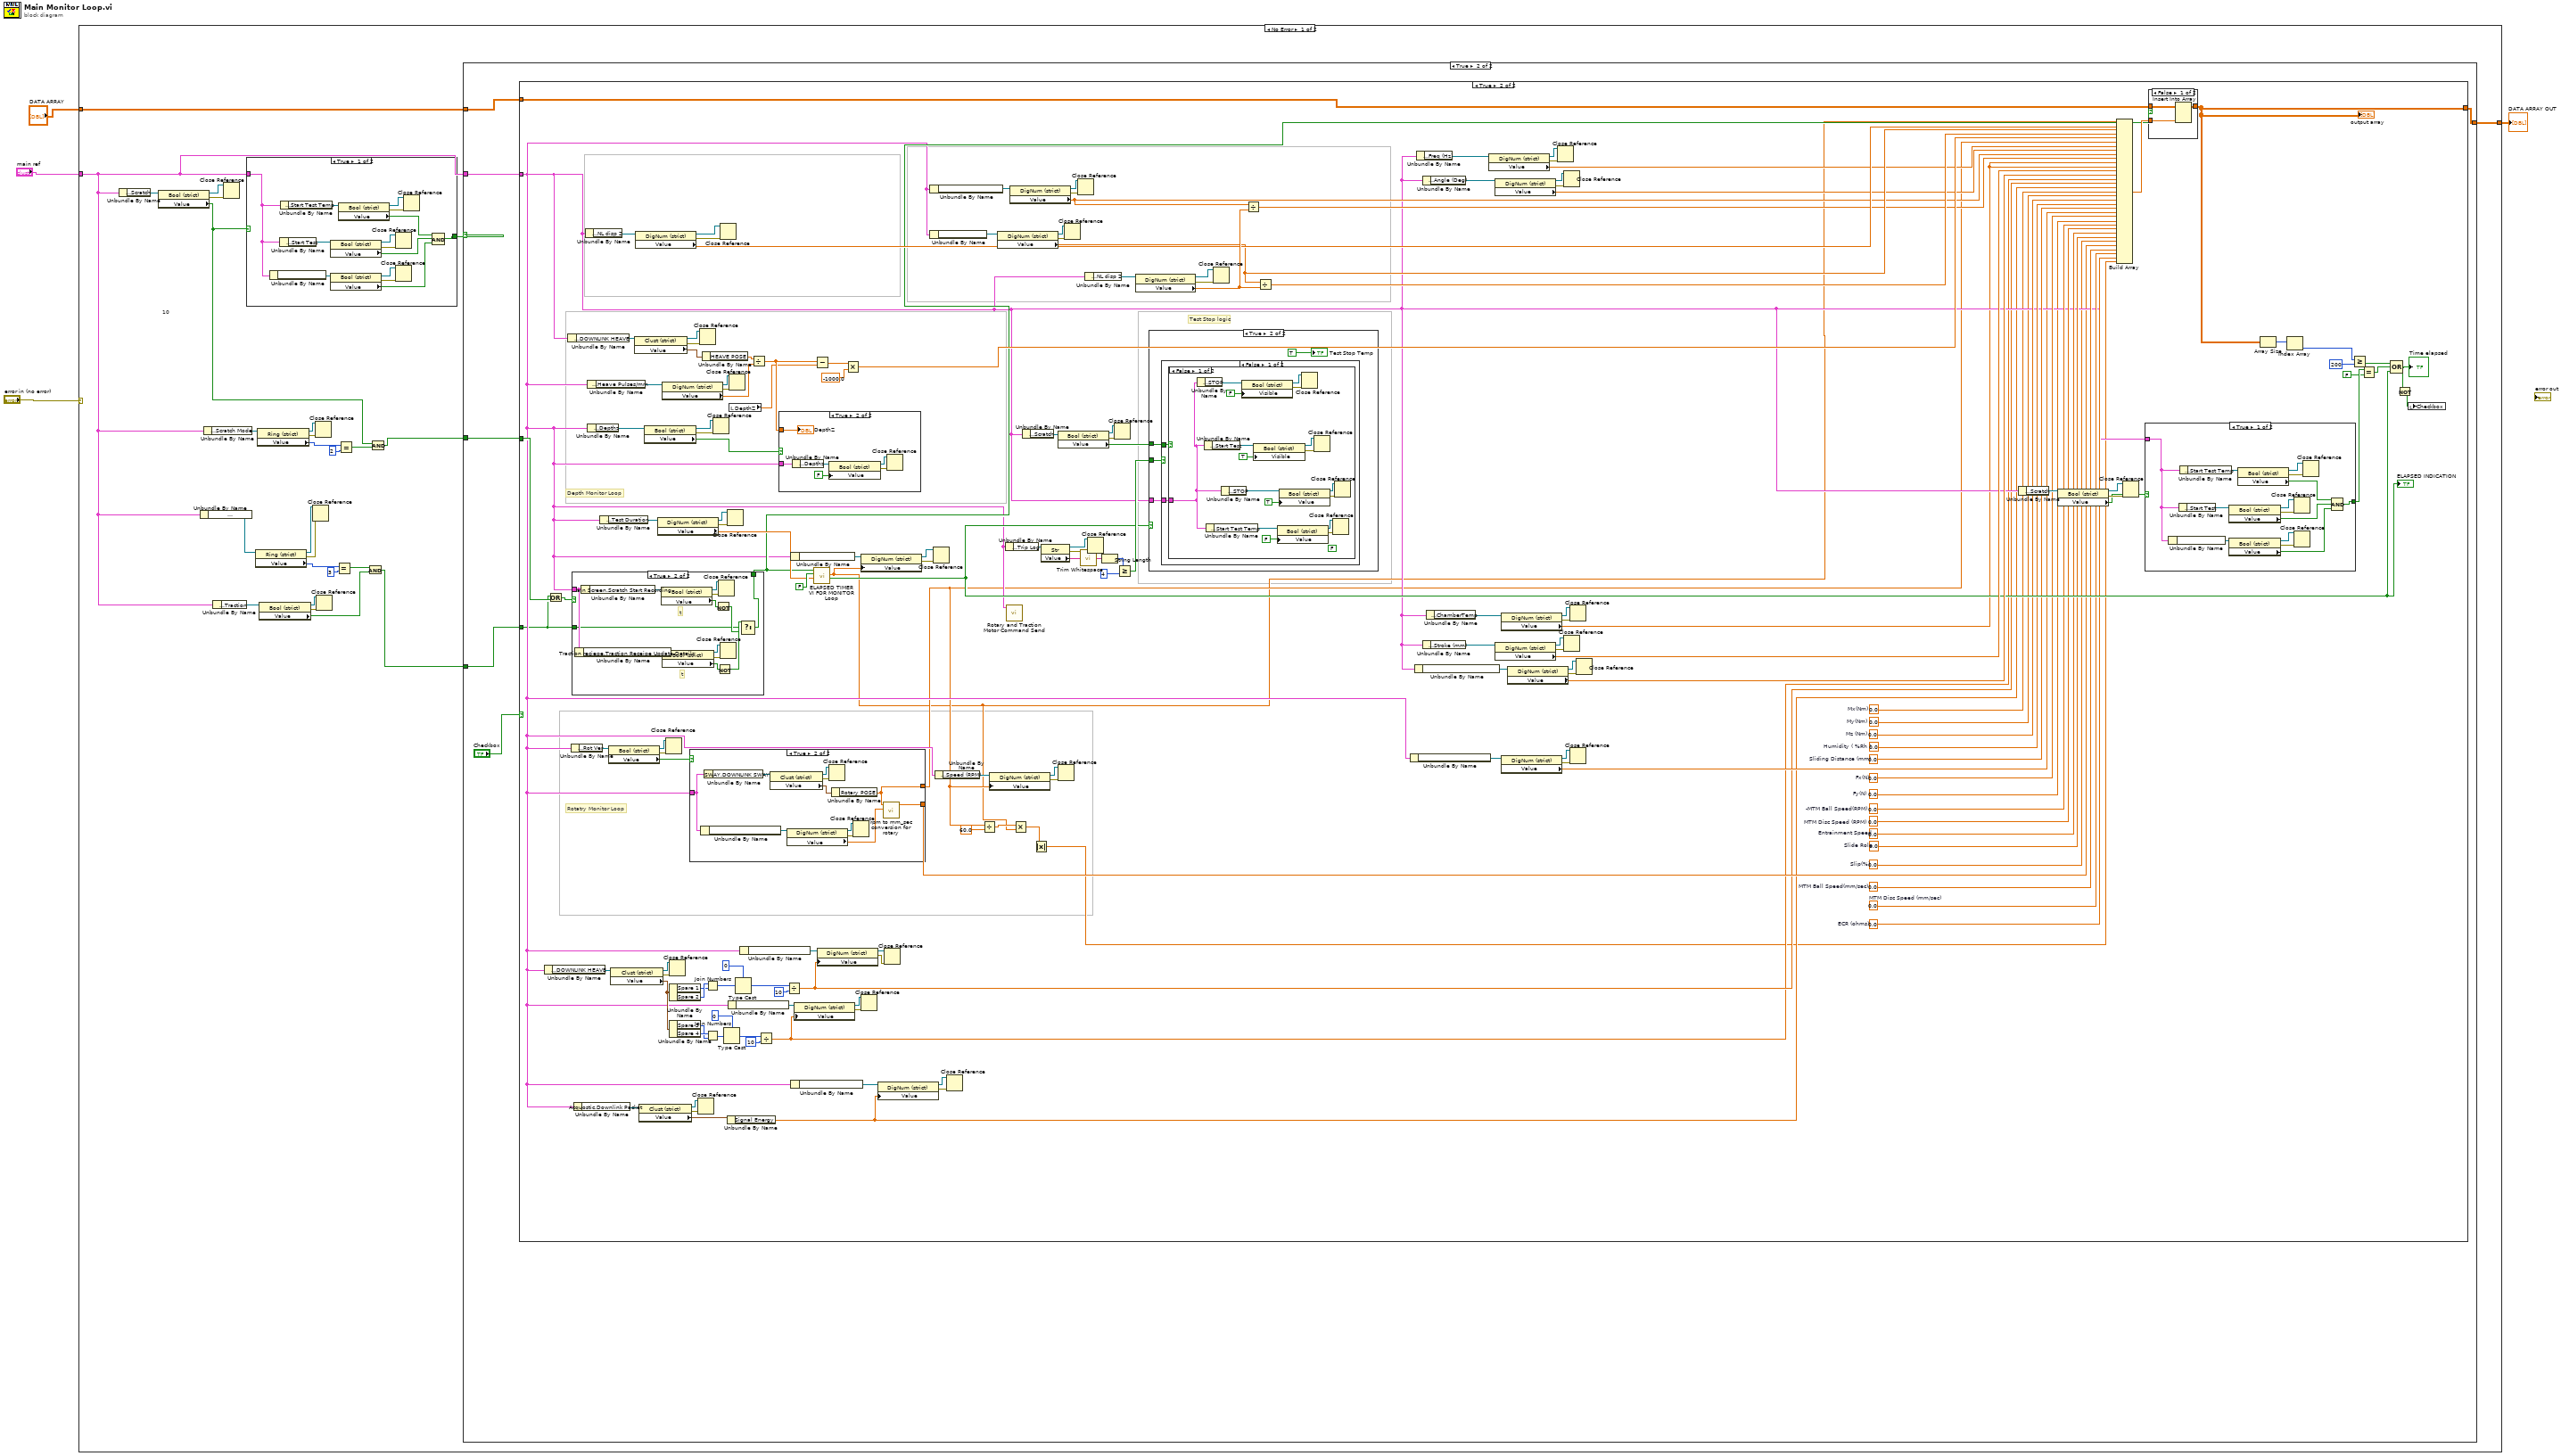
[diagram p0: block diagram]
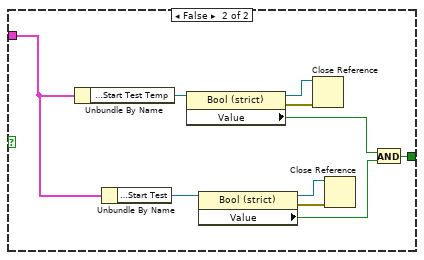
[diagram p2: hidden frame]
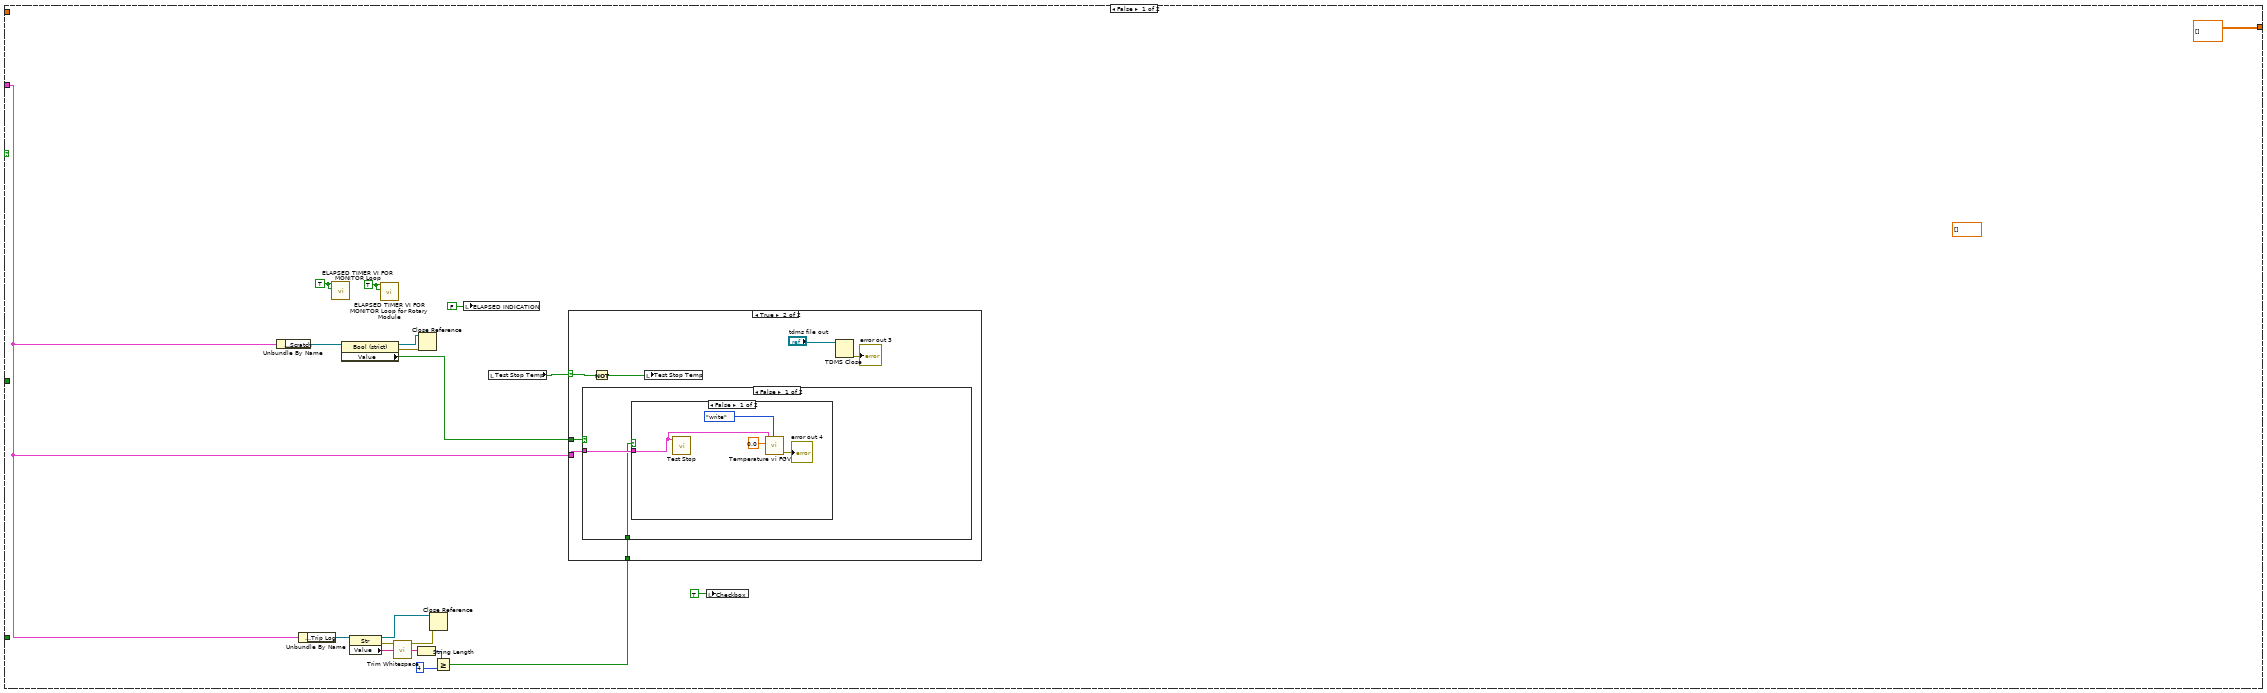
[diagram p3: hidden frame]
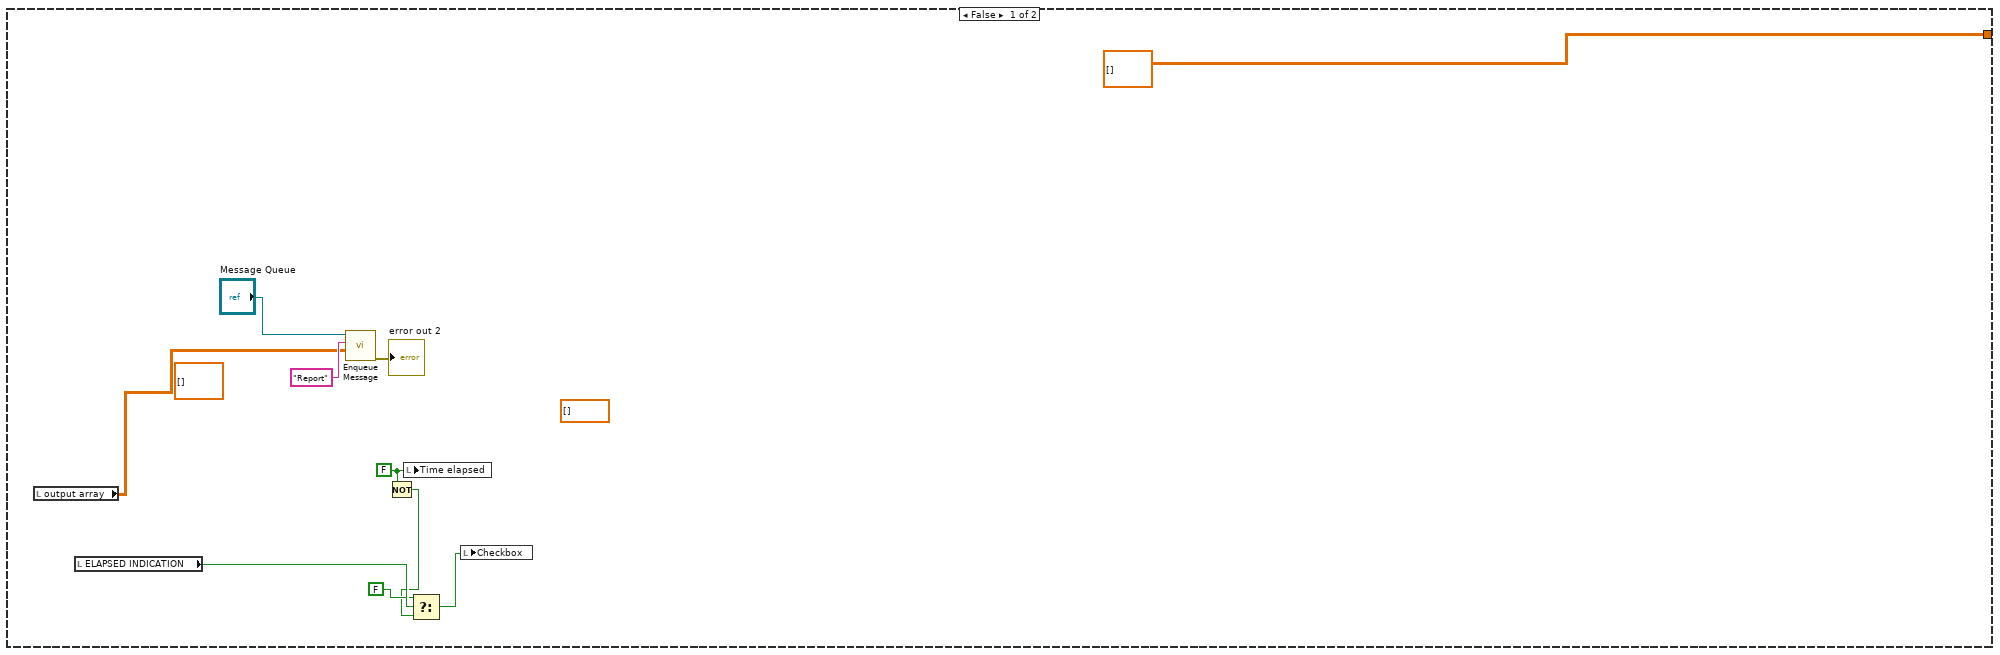
[diagram p7: hidden frame]
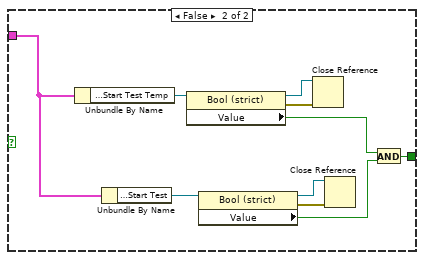
[diagram p9: hidden frame]
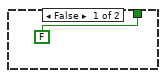
[diagram p10: hidden frame]
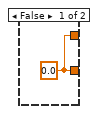
[diagram p11: hidden frame]
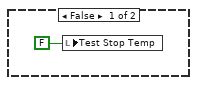
[diagram p12: hidden frame]
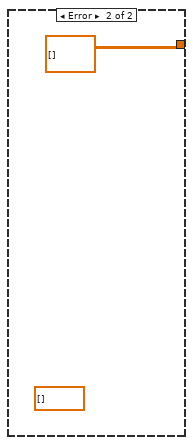
[diagram p16: hidden frame]
diagram:
  n1 = case shown="No Error" "error in (no error)" {
    tunnel: "main ref" -> [w7 _]
    tunnel: "DATA ARRAY" -> [w18 _]
    tunnel: [w17 dbl[][] [] ("DATA ARRAY")] -> w1
    frame No Error {
      # "10"
      n2 = Unbundle By Name(w7) -> ("Motion Module.Scratch"=w28:refnum<vi>)
      n3 = property class="Bool (strict)"(reference=w28) -> (reference out=w29:refnum<vi>, error out=w27:errorcluster, "Value"=w20:bool)  [unwired: 1 in]
      n4 = Unbundle By Name(w7) -> ("Traction Control.Motion Mode:"=w15:refnum<vi>)
      n5 = Unbundle By Name(w7) -> ("Motion Module.Scratch Mode"=w22:refnum<vi>)
      n6 = Unbundle By Name(w7) -> ("Motion Module.Traction"=w9:refnum<vi>)
      n7 = Close Reference(reference=w29, error in (no error)=w27) -> ()  [unwired: 1 out]
      n8 = case shown="True" w20 {
        tunnel: w7 -> [w32 w48]
        tunnel: [w36 w46] -> w30
        frame True {
          n9 = Unbundle By Name(w32) -> ("Main Screen.Scratch Start Test"=w34:refnum<vi>)
          n10 = Unbundle By Name(w32) -> ("Main Screen.Start Test"=w40:refnum<vi>)
          n11 = Unbundle By Name(w32) -> ("Main Screen.Start Test Temp"=w43:refnum<vi>)
          n12 = property class="Bool (strict)"(reference=w40) -> (reference out=w39:refnum<vi>, error out=w41:errorcluster, "Value"=w37:bool)  [unwired: 1 in]
          n13 = property class="Bool (strict)"(reference=w34) -> (reference out=w35:refnum<vi>, error out=w33:errorcluster, "Value"=w31:bool)  [unwired: 1 in]
          n14 = property class="Bool (strict)"(reference=w43) -> (reference out=w44:refnum<vi>, error out=w42:errorcluster, "Value"=w38:bool)  [unwired: 1 in]
          n15 = Close Reference(reference=w39, error in (no error)=w41) -> ()  [unwired: 1 out]
          n16 = Close Reference(reference=w35, error in (no error)=w33) -> ()  [unwired: 1 out]
          n17 = Close Reference(reference=w44, error in (no error)=w42) -> ()  [unwired: 1 out]
          n18 = Compound Arithmetic op=AND(w38, w37, w31) -> (w36:bool)
        }
        frame False {
          n19 = Unbundle By Name(w48) -> ("Main Screen.Start Test Temp"=w53:refnum<vi>)
          n20 = Unbundle By Name(w48) -> ("Main Screen.Start Test"=w50:refnum<vi>)
          n21 = property class="Bool (strict)"(reference=w53) -> (reference out=w54:refnum<vi>, error out=w52:errorcluster, "Value"=w47:bool)  [unwired: 1 in]
          n22 = property class="Bool (strict)"(reference=w50) -> (reference out=w49:refnum<vi>, error out=w51:errorcluster, "Value"=w45:bool)  [unwired: 1 in]
          n23 = Close Reference(reference=w54, error in (no error)=w52) -> ()  [unwired: 1 out]
          n24 = Close Reference(reference=w49, error in (no error)=w51) -> ()  [unwired: 1 out]
          n25 = And(x=w47, y=w45) -> (x .and. y?=w46:bool)
        }
      }
      n26 = property class="Ring (strict)"(reference=w15) -> (reference out=w16:refnum<vi>, error out=w14:errorcluster, "Value"=w13:u16)  [unwired: 1 in]
      n27 = property class="Ring (strict)"(reference=w22) -> (reference out=w21:refnum<vi>, error out=w23:errorcluster, "Value"=w24:u16)  [unwired: 1 in]
      n28 = property class="Bool (strict)"(reference=w9) -> (reference out=w8:refnum<vi>, error out=w10:errorcluster, "Value"=w6:bool)  [unwired: 1 in]
      n29 = Close Reference(reference=w16, error in (no error)=w14) -> ()  [unwired: 1 out]
      n30 = Close Reference(reference=w21, error in (no error)=w23) -> ()  [unwired: 1 out]
      n31 = Close Reference(reference=w8, error in (no error)=w10) -> ()  [unwired: 1 out]
      n32 = Equal?(x=w13, y=u16 3) -> (x = y?=w11:bool)
      n33 = Equal?(x=w24, y=u16 2) -> (x = y?=w26:bool)
      n34 = Compound Arithmetic op=AND(w11, w6) -> (w5:bool)
      n35 = Compound Arithmetic op=AND(w20, w26) -> (w19:bool)
      n36 = case shown="True" w30 {
        tunnel: w7 -> [w58 w91]
        tunnel: w19 -> [_ w92]
        tunnel: w18 -> [_ w90]
        tunnel: [dbl[][] [] ("DATA ARRAY") w89] -> w17
        tunnel: w5 -> [_ w87]
        frame False {
          (unwired) dbl[] [] ("DATA ARRAY")
          w67 = TRUE ("PAUSE")
          w73 = TRUE ("PAUSE")
          n37 = Unbundle By Name(w58) -> ("Motion Module.Scratch"=w71:refnum<vi>)
          n38 = Unbundle By Name(w58) -> ("Main Screen.Trip Log"=w65:refnum<vi>)
          n39 = call "ELAPSED TIMER VI FOR MONITOR Loop.vi"("RESET"=w73, "PAUSE"=w73) -> ()  [unwired: 7 in, 3 out]
          n40 = property class="Bool (strict)"(reference=w71) -> (reference out=w69:refnum<vi>, error out=w70:errorcluster, "Value"=w68:bool)  [unwired: 1 in]
          n41 = property class="Str"(reference=w65) -> (reference out=w60:refnum<vi>, error out=w66:errorcluster, "Value"=w64:string)  [unwired: 1 in]
          n42 = call "ELAPSED TIMER VI FOR MONITOR Loop for Rotary Module.vi"("RESET"=w67, "PAUSE"=w67) -> ()  [unwired: 7 in, 3 out]
          n43 = call <vilib>:"Trim Whitespace.vi"("string"=w64) -> ("trimmed string"=w63:string)  [unwired: 1 in]
          n44 = String Length(string=w63) -> (length=w62:i32)
          n45 = Close Reference(reference=w69, error in (no error)=w70) -> ()  [unwired: 1 out]
          n46 = Close Reference(reference=w60, error in (no error)=w66) -> ()  [unwired: 1 out]
          n47 = Greater Or Equal?(x=w62, y=4) -> (x >= y?=w59:bool)
          n48 = local write "ELAPSED INDICATION"(FALSE ("ELAPSED INDICATION")) -> ()
          n49 = local read "Test Stop Temp"() -> (w72:bool)
          n50 = case shown="True" w72 {
            selector: w72 -> [_ w80]
            tunnel: w58 -> [_ w78]
            tunnel: w68 -> [_ w77]
            tunnel: w59 -> [_ w76]
            frame False {
            }
            frame True {
              n51 = case shown="False" w77 {
                tunnel: w78 -> [w82 _]
                tunnel: w76 -> [w81 _]
                frame False {
                  n52 = case shown="False" w81 {
                    tunnel: w82 -> [w84 _]
                    frame False {
                      n53 = call "Test Stop.vi"("Data Cluster"=w84) -> ()  [unwired: 10 in, 1 out]
                      n54 = call "Temperature vi FGV.vi"("Enum"=Temperature_enum."write", "Set Temperature"=0.0, "main ref"=w84) -> ("error out"=→"error out 4":errorcluster)  [unwired: 8 in]
                    }
                    frame True {
                    }
                  }
                }
                frame True {
                }
              }
              n55 = Not(x=w80) -> (.not. x?=w79:bool)
              n56 = local write "Test Stop Temp"(w79) -> ()
              n57 = TDMS Close(11:"tdms file out") -> (0:→"error out 3":errorcluster)  [unwired: 1 in, 1 out]
            }
          }
          n58 = local write "Checkbox"(TRUE ("Checkbox")) -> ()
        }
        frame True {
          n59 = case shown="True" "Checkbox" {
            tunnel: w92 -> [_ w179]
            tunnel: w91 -> [_ w121]
            tunnel: w90 -> [_ w178]
            tunnel: [dbl[][] [] ("DATA ARRAY") w135] -> w89
            tunnel: w87 -> [_ w119]
            frame False {
              (unwired) dbl[][] [] ("output data")
              w99 = FALSE ("Time elapsed")
              (unwired) dbl[] [] ("DATA ARRAY")
              n60 = local read "output array"() -> (w97:dbl[][])
              n61 = local read "ELAPSED INDICATION"() -> (w96:bool)
              n62 = call-poly "Enqueue Message.vi"("output data"=w97, "Message"="Report", "Message Queue"="Message Queue") -> ("error out"=→"error out 2":errorcluster)  [unwired: 7 in, 1 out]
              n63 = Not(x=w99) -> (.not. x?=w93:bool)
              n64 = local write "Time elapsed"(w99) -> ()
              n65 = Select(t=FALSE, s=w96, f=w93) -> (s? t:f=w94:bool)
              n66 = local write "Checkbox"(w94) -> ()
            }
            frame True {
              w108 = 0.0  # Mx(Nm)
              w111 = 0.0  # Fy(N)
              w123 = 0.0  # ECR (ohms)
              w124 = 0.0  # MTM Disc Speed (mm/sec)
              w125 = 0.0  # MTM Ball Speed(mm/sec)
              w113 = 0.0  # Slip(%)
              w109 = 0.0  # My(Nm)
              w128 = 0.0  # MTM Disc Speed (RPM)
              w129 = 0.0  # -MTM Ball Speed(RPM)
              w126 = 0.0  # Slide Role
              w127 = 0.0  # Entrainment Speed
              w131 = 0.0  # Sliding Distance (mm)
              w132 = 0.0  # Humidity ( %Rh )
              w133 = 0.0  # Mz (Nm)
              w130 = 0.0  # Fx(N)
              # "Rotatry Monitor Loop"
              # "Test Stop logic"
              # "Depth Monitor Loop"
              n67 = Unbundle By Name(w121) -> ("Heave AND Surge.DOWNLINK HEAVE"=w208:refnum<vi>)
              n68 = Or(x=w119, y=w179) -> (x .or. y?=w120:bool)
              n69 = Unbundle By Name(w121) -> ("Heave AND Surge.DOWNLINK HEAVE"=w215:refnum<vi>)
              n70 = Unbundle By Name(w121) -> ("Motion Module.Rot Ver"=w228:refnum<vi>)
              n71 = case shown="True" w120 {
                tunnel: w121 -> [_ w300]
                tunnel: [FALSE ("Value") w296] -> w122
                tunnel: w119 -> [_ w297]
                frame False {
                }
                frame True {
                  # "t"
                  # "t"
                  n72 = Unbundle By Name(w300) -> ("Traction reciepe.Traction Receipe Update Details"=w302:refnum<vi>)
                  n73 = Unbundle By Name(w300) -> ("Main Screen.Scratch Start Recording"=w306:refnum<vi>)
                  n74 = property class="Bool (strict)"(reference=w306) -> (reference out=w305:refnum<vi>, error out=w307:errorcluster, "Value"=w304:bool)  [unwired: 1 in]
                  n75 = property class="Bool (strict)"(reference=w302) -> (reference out=w295:refnum<vi>, error out=w301:errorcluster, "Value"=w303:bool)  [unwired: 1 in]
                  n76 = Not(x=w304) -> (.not. x?=w298:bool)
                  n77 = Not(x=w303) -> (.not. x?=w299:bool)
                  n78 = Close Reference(reference=w305, error in (no error)=w307) -> ()  [unwired: 1 out]
                  n79 = Close Reference(reference=w295, error in (no error)=w301) -> ()  [unwired: 1 out]
                  n80 = Select(t=w299, s=w297, f=w298) -> (s? t:f=w296:bool)
                }
              }
              n81 = Unbundle By Name(w121) -> ("Acquostic.Downlink Packet"=w186:refnum<vi>)
              n82 = Unbundle By Name(w121) -> ("Main Screen.NL disp 2"=w265:refnum<vi>)
              n83 = Unbundle By Name(w121) -> ("Config Parameters.Heave Pulses/mm"=w261:refnum<vi>)
              n84 = Unbundle By Name(w121) -> ("Main Screen.Depthz"=w257:refnum<vi>)
              n85 = Unbundle By Name(w121) -> ("Main Screen.Test Duration"=w248:refnum<vi>)
              n86 = property class="Bool (strict)"(reference=w228) -> (reference out=w226:refnum<vi>, error out=w227:errorcluster, "Value"=w225:bool)  [unwired: 1 in]
              n87 = property class="Clust (strict)"(reference=w208) -> (reference out=w206:refnum<vi>, error out=w207:errorcluster, "Value"=w205:T3)  [unwired: 1 in]
              n88 = property on="Property Node" class="Clust (strict)"(reference=w215) -> (reference out=w217:refnum<vi>, error out=w216:errorcluster, "Value"=w214:T3)  [unwired: 1 in]
              n89 = property class="DigNum (strict)"(reference=w265) -> (reference out=w263:refnum<vi>, error out=w264:errorcluster, "Value"=w177:dbl)  [unwired: 1 in]
              n90 = property on="Property Node" class="Clust (strict)"(reference=w186) -> (reference out=w184:refnum<vi>, error out=w185:errorcluster, "Value"=w183:T4)  [unwired: 1 in]
              n91 = property class="Bool (strict)"(reference=w257) -> (reference out=w258:refnum<vi>, error out=w256:errorcluster, "Value"=w255:bool)  [unwired: 1 in]
              n92 = property class="DigNum (strict)"(reference=w248) -> (reference out=w249:refnum<vi>, error out=w247:errorcluster, "Value"=w246:dbl)  [unwired: 1 in]
              n93 = property class="DigNum (strict)"(reference=w261) -> (reference out=w260:refnum<vi>, error out=w262:errorcluster, "Value"=w259:dbl)  [unwired: 1 in]
              n94 = Close Reference(reference=w226, error in (no error)=w227) -> ()  [unwired: 1 out]
              n95 = Close Reference(reference=w206, error in (no error)=w207) -> ()  [unwired: 1 out]
              n96 = Unbundle By Name(w205) -> ("Spare 1"=w195:u8, "Spare 2"=w196:u8)
              n97 = Unbundle By Name(w205) -> ("Spare 3"=w188:u8, "Spare 4"=w189:u8)
              n98 = case shown="True" w225 {
                tunnel: w121 -> [_ w310]
                tunnel: [w308 w315] -> w112
                tunnel: [w308 w309] -> w118
                frame False {
                  w308 = 0.0 ("Enter initial Velocity (m/s)  4")
                }
                frame True {
                  n99 = Unbundle By Name(w310) -> ("Motion Module.Wear Track Diameter (mm)"=w319:refnum<vi>)
                  n100 = Unbundle By Name(w310) -> ("SWAY.DOWNLINK SWAY"=w312:refnum<vi>)
                  n101 = property on="Property Node" class="Clust (strict)"(reference=w312) -> (reference out=w314:refnum<vi>, error out=w313:errorcluster, "Value"=w311:T5)  [unwired: 1 in]
                  n102 = property class="DigNum (strict)"(reference=w319) -> (reference out=w317:refnum<vi>, error out=w318:errorcluster, "Value"=w316:dbl)  [unwired: 1 in]
                  n103 = Close Reference(reference=w314, error in (no error)=w313) -> ()  [unwired: 1 out]
                  n104 = Unbundle By Name(w311) -> ("Rotary POSE"=w309:sgl)
                  n105 = Close Reference(reference=w317, error in (no error)=w318) -> ()  [unwired: 1 out]
                  n106 = call "rpm to mm_sec conversion for rotary.vi"("Wear Track Diameter"=w316, "Initial Speed (RPM)"=w309) -> ("Enter initial Velocity (m/s)  4"=w315:dbl)  [unwired: 7 in, 2 out]
                }
              }
              n107 = Close Reference(reference=w184, error in (no error)=w185) -> ()  [unwired: 1 out]
              n108 = Close Reference(reference=w217, error in (no error)=w216) -> ()  [unwired: 1 out]
              n109 = Unbundle By Name(w214) -> ("HEAVE POSE"=w213:sgl)
              n110 = Join Numbers(hi=w196, lo=w195) -> ((hi.lo)=w193:u16)
              n111 = Join Numbers(hi=w189, lo=w188) -> ((hi.lo)=w190:u16)
              n112 = Close Reference(reference=w258, error in (no error)=w256) -> ()  [unwired: 1 out]
              n113 = Close Reference(reference=w263, error in (no error)=w264) -> ()  [unwired: 1 out]
              n114 = Type Cast(type=i16 0, x=w190) -> (*(type *) &x=w187:i16)
              n115 = Close Reference(reference=w249, error in (no error)=w247) -> ()  [unwired: 1 out]
              n116 = Unbundle By Name(w183) -> ("Signal Energy"=w107:sgl)
              n117 = Unbundle By Name(w121) -> ("Main Screen.Ambient\n Humidity"=w201:refnum<vi>)
              n118 = Close Reference(reference=w260, error in (no error)=w262) -> ()  [unwired: 1 out]
              n119 = local read "DepthZ"() -> (w253:dbl)
              n120 = Type Cast(type=i16 0, x=w193) -> (*(type *) &x=w192:i16)
              n121 = Unbundle By Name(w121) -> ("Main Screen.Ambient \nTemperature"=w204:refnum<vi>)
              n122 = Divide(x=w213, y=w259) -> (x/y=w254:dbl)
              n123 = Divide(x=w187, y=u8 10) -> (x/y=w105:dbl)
              n124 = case shown="True" w255 {
                tunnel: w254 -> [_ w349]
                tunnel: w121 -> [_ w345]
                frame False {
                }
                frame True {
                  n125 = Unbundle By Name(w345) -> ("Main Screen.Depthz"=w347:refnum<vi>)
                  n126 = property class="Bool (strict)"(reference=w347, "Value"=FALSE) -> (reference out=w346:refnum<vi>, error out=w348:errorcluster)  [unwired: 1 in]
                  n127 = Close Reference(reference=w346, error in (no error)=w348) -> ()  [unwired: 1 out]
                  "DepthZ" <- w349
                }
              }
              n128 = Divide(x=w192, y=u8 10) -> (x/y=w106:dbl)
              n129 = Unbundle By Name(w121) -> ("Main Screen.Time ( HH:MM:SS ) 2"=w230:refnum<vi>)
              n130 = Unbundle By Name(w121) -> ("Main Screen.Acoustic Emission (mV)"=w181:refnum<vi>)
              n131 = property class="DigNum (strict)"(reference=w201, "Value"=w105) -> (reference out=w197:refnum<vi>, error out=w200:errorcluster)  [unwired: 1 in]
              n132 = call "ELAPSED TIMER VI FOR MONITOR Loop.vi"("TARGET"=w246, "RESET"=FALSE ("PAUSE"), "PAUSE"=w122) -> ("ELAPSED INDICATION"=w140:bool, "ELAPSED TIMER"=w115:dbl)  [unwired: 6 in, 1 out]
              "ELAPSED INDICATION" <- w140
              n133 = Subtract(x=w254, y=w253) -> (x-y=w252:dbl)
              n134 = property class="DigNum (strict)"(reference=w204, "Value"=w106) -> (reference out=w198:refnum<vi>, error out=w203:errorcluster)  [unwired: 1 in]
              n135 = Multiply(x=w252, y=-1000.0) -> (x*y=w174:dbl)
              n136 = property class="DigNum (strict)"(reference=w230, "Value"=w115) -> (reference out=w244:refnum<vi>, error out=w245:errorcluster)  [unwired: 1 in]
              n137 = Close Reference(reference=w197, error in (no error)=w200) -> ()  [unwired: 1 out]
              n138 = property class="DigNum (strict)"(reference=w181, "Value"=w107) -> (reference out=w180:refnum<vi>, error out=w182:errorcluster)  [unwired: 1 in]
              n139 = Close Reference(reference=w198, error in (no error)=w203) -> ()  [unwired: 1 out]
              n140 = Unbundle By Name(w121) -> ("Main Screen.Cyclic Friction Force (N)"=w240:refnum<vi>)
              n141 = Unbundle By Name(w121) -> ("Main Screen.Friction Force (N)"=w242:refnum<vi>)
              n142 = Close Reference(reference=w244, error in (no error)=w245) -> ()  [unwired: 1 out]
              n143 = Unbundle By Name(w121) -> ("Main Screen.Speed (RPM)"=w224:refnum<vi>)
              n144 = Close Reference(reference=w180, error in (no error)=w182) -> ()  [unwired: 1 out]
              n145 = Divide(x=w118, y=60.0) -> (x/y=w116:dbl)
              n146 = property class="DigNum (strict)"(reference=w224, "Value"=w118) -> (reference out=w222:refnum<vi>, error out=w223:errorcluster)  [unwired: 1 in]
              n147 = property class="DigNum (strict)"(reference=w242) -> (reference out=w243:refnum<vi>, error out=w241:errorcluster, "Value"=w176:dbl)  [unwired: 1 in]
              n148 = Unbundle By Name(w121) -> ("Main Screen.Trip Log"=w219:refnum<vi>)
              n149 = call "Rotary and Traction Motor Command Send.vi"("main ref"=w121) -> ()  [unwired: 10 in, 1 out]
              n150 = property class="DigNum (strict)"(reference=w240) -> (reference out=w238:refnum<vi>, error out=w239:errorcluster, "Value"=w165:dbl)  [unwired: 1 in]
              n151 = Multiply(x=w116, y=w115) -> (x*y=w114:dbl)
              n152 = Unbundle By Name(w121) -> ("Motion Module.Scratch"=w229:refnum<vi>)
              n153 = Absolute Value(x=w114) -> (abs(x)=w103:dbl)
              n154 = property class="Str"(reference=w219) -> (reference out=w221:refnum<vi>, error out=w220:errorcluster, "Value"=w218:string)  [unwired: 1 in]
              n155 = property class="Bool (strict)"(reference=w229) -> (reference out=w236:refnum<vi>, error out=w237:errorcluster, "Value"=w235:bool)  [unwired: 1 in]
              n156 = Close Reference(reference=w222, error in (no error)=w223) -> ()  [unwired: 1 out]
              n157 = Close Reference(reference=w243, error in (no error)=w241) -> ()  [unwired: 1 out]
              n158 = Close Reference(reference=w238, error in (no error)=w239) -> ()  [unwired: 1 out]
              n159 = call <vilib>:"Trim Whitespace.vi"("string"=w218) -> ("trimmed string"=w212:string)  [unwired: 1 in]
              n160 = Unbundle By Name(w121) -> ("Main Screen.NL disp 2"=w234:refnum<vi>)
              n161 = Close Reference(reference=w221, error in (no error)=w220) -> ()  [unwired: 1 out]
              n162 = String Length(string=w212) -> (length=w211:i32)
              n163 = Close Reference(reference=w236, error in (no error)=w237) -> ()  [unwired: 1 out]
              n164 = Greater Or Equal?(x=w211, y=4) -> (x >= y?=w209:bool)
              n165 = property class="DigNum (strict)"(reference=w234) -> (reference out=w232:refnum<vi>, error out=w233:errorcluster, "Value"=w231:dbl)  [unwired: 1 in]
              n166 = case shown="True" w140 {
                tunnel: w121 -> [_ w323]
                tunnel: w235 -> [_ w322]
                tunnel: w209 -> [_ w321]
                frame False {
                  n167 = local write "Test Stop Temp"(FALSE ("Test Stop Temp")) -> ()
                }
                frame True {
                  n168 = case shown="False" w321 {
                    tunnel: w323 -> [w326 _]
                    tunnel: w322 -> [w325 _]
                    frame False {
                      n169 = case shown="False" w325 {
                        tunnel: w326 -> [w327 _]
                        frame False {
                          (unwired) FALSE ("y")
                          n170 = Unbundle By Name(w327) -> ("Main Screen.STOP"=w333:refnum<vi>)
                          n171 = Unbundle By Name(w327) -> ("Main Screen.Start Test"=w330:refnum<vi>)
                          n172 = Unbundle By Name(w327) -> ("Main Screen.Start Test Temp"=w341:refnum<vi>)
                          n173 = Unbundle By Name(w327) -> ("Main Screen.STOP"=w340:refnum<vi>)
                          n174 = property class="Bool (strict)"(reference=w333, "Visible"=FALSE) -> (reference out=w335:refnum<vi>, error out=w334:errorcluster)  [unwired: 1 in]
                          n175 = property class="Bool (strict)"(reference=w330, "Visible"=TRUE) -> (reference out=w328:refnum<vi>, error out=w329:errorcluster)  [unwired: 1 in]
                          n176 = property class="Bool (strict)"(reference=w341, "Value"=FALSE) -> (reference out=w343:refnum<vi>, error out=w342:errorcluster)  [unwired: 1 in]
                          n177 = property class="Bool (strict)"(reference=w340, "Value"=TRUE) -> (reference out=w338:refnum<vi>, error out=w339:errorcluster)  [unwired: 1 in]
                          n178 = Close Reference(reference=w335, error in (no error)=w334) -> ()  [unwired: 1 out]
                          n179 = Close Reference(reference=w328, error in (no error)=w329) -> ()  [unwired: 1 out]
                          n180 = Close Reference(reference=w343, error in (no error)=w342) -> ()  [unwired: 1 out]
                          n181 = Close Reference(reference=w338, error in (no error)=w339) -> ()  [unwired: 1 out]
                        }
                        frame True {
                        }
                      }
                    }
                    frame True {
                    }
                  }
                  "Test Stop Temp" <- TRUE ("Test Stop Temp")
                }
              }
              n182 = Close Reference(reference=w232, error in (no error)=w233) -> ()  [unwired: 1 out]
              n183 = Divide(x=w165, y=w231) -> (x/y=w164:dbl)
              n184 = Divide(x=w176, y=w231) -> (x/y=w175:dbl)
              n185 = Unbundle By Name(w121) -> ("Motion Module.Wear Track Diameter (mm)"=w151:refnum<vi>)
              n186 = Unbundle By Name(w121) -> ("Motion Module.Enter Scratch Speed (mm/s):"=w156:refnum<vi>)
              n187 = Unbundle By Name(w121) -> ("Main Screen.Freq (Hz)"=w172:refnum<vi>)
              n188 = Unbundle By Name(w121) -> ("Main Screen.Angle (Deg)"=w171:refnum<vi>)
              n189 = Unbundle By Name(w121) -> ("Main Screen.Stroke (mm)"=w159:refnum<vi>)
              n190 = Unbundle By Name(w121) -> ("Main Screen.ChamberTemp"=w162:refnum<vi>)
              n191 = property class="DigNum (strict)"(reference=w172) -> (reference out=w168:refnum<vi>, error out=w173:errorcluster, "Value"=w167:dbl)  [unwired: 1 in]
              n192 = property class="DigNum (strict)"(reference=w171) -> (reference out=w169:refnum<vi>, error out=w170:errorcluster, "Value"=w166:dbl)  [unwired: 1 in]
              n193 = property class="DigNum (strict)"(reference=w159) -> (reference out=w160:refnum<vi>, error out=w158:errorcluster, "Value"=w154:dbl)  [unwired: 1 in]
              n194 = property class="DigNum (strict)"(reference=w162) -> (reference out=w161:refnum<vi>, error out=w163:errorcluster, "Value"=w104:dbl)  [unwired: 1 in]
              n195 = property class="DigNum (strict)"(reference=w151) -> (reference out=w150:refnum<vi>, error out=w152:errorcluster, "Value"=w110:dbl)  [unwired: 1 in]
              n196 = property class="DigNum (strict)"(reference=w156) -> (reference out=w155:refnum<vi>, error out=w157:errorcluster, "Value"=w153:dbl)  [unwired: 1 in]
              n197 = Close Reference(reference=w168, error in (no error)=w173) -> ()  [unwired: 1 out]
              n198 = Close Reference(reference=w169, error in (no error)=w170) -> ()  [unwired: 1 out]
              n199 = Close Reference(reference=w160, error in (no error)=w158) -> ()  [unwired: 1 out]
              n200 = Close Reference(reference=w161, error in (no error)=w163) -> ()  [unwired: 1 out]
              n201 = Close Reference(reference=w150, error in (no error)=w152) -> ()  [unwired: 1 out]
              n202 = Close Reference(reference=w155, error in (no error)=w157) -> ()  [unwired: 1 out]
              n203 = Unbundle By Name(w121) -> ("Motion Module.Scratch"=w147:refnum<vi>)
              n204 = property class="Bool (strict)"(reference=w147) -> (reference out=w148:refnum<vi>, error out=w146:errorcluster, "Value"=w145:bool)  [unwired: 1 in]
              n205 = Build Array(w115, w177, w176, w175, w174, w118, w167, w166, w165, w164, w104, w104, w154, w153, w105, w106, w107, w108, w109, w133, w132, w131, w110, w130, w111, w129, w128, w127, w126, w113, w112, w125, w124, w123, w103) -> (w136:dbl[])
              n206 = Close Reference(reference=w148, error in (no error)=w146) -> ()  [unwired: 1 out]
              n207 = case shown="True" w145 {
                tunnel: w121 -> [w271 w287]
                tunnel: [w275 w285] -> w144
                frame True {
                  n208 = Unbundle By Name(w271) -> ("Main Screen.Scratch Start Test"=w273:refnum<vi>)
                  n209 = Unbundle By Name(w271) -> ("Main Screen.Start Test"=w279:refnum<vi>)
                  n210 = Unbundle By Name(w271) -> ("Main Screen.Start Test Temp"=w282:refnum<vi>)
                  n211 = property class="Bool (strict)"(reference=w279) -> (reference out=w278:refnum<vi>, error out=w280:errorcluster, "Value"=w276:bool)  [unwired: 1 in]
                  n212 = property class="Bool (strict)"(reference=w273) -> (reference out=w274:refnum<vi>, error out=w272:errorcluster, "Value"=w270:bool)  [unwired: 1 in]
                  n213 = property class="Bool (strict)"(reference=w282) -> (reference out=w283:refnum<vi>, error out=w281:errorcluster, "Value"=w277:bool)  [unwired: 1 in]
                  n214 = Close Reference(reference=w278, error in (no error)=w280) -> ()  [unwired: 1 out]
                  n215 = Close Reference(reference=w274, error in (no error)=w272) -> ()  [unwired: 1 out]
                  n216 = Close Reference(reference=w283, error in (no error)=w281) -> ()  [unwired: 1 out]
                  n217 = Compound Arithmetic op=AND(w277, w276, w270) -> (w275:bool)
                }
                frame False {
                  n218 = Unbundle By Name(w287) -> ("Main Screen.Start Test Temp"=w292:refnum<vi>)
                  n219 = Unbundle By Name(w287) -> ("Main Screen.Start Test"=w289:refnum<vi>)
                  n220 = property class="Bool (strict)"(reference=w292) -> (reference out=w293:refnum<vi>, error out=w291:errorcluster, "Value"=w286:bool)  [unwired: 1 in]
                  n221 = property class="Bool (strict)"(reference=w289) -> (reference out=w288:refnum<vi>, error out=w290:errorcluster, "Value"=w284:bool)  [unwired: 1 in]
                  n222 = Close Reference(reference=w293, error in (no error)=w291) -> ()  [unwired: 1 out]
                  n223 = Close Reference(reference=w288, error in (no error)=w290) -> ()  [unwired: 1 out]
                  n224 = And(x=w286, y=w284) -> (x .and. y?=w285:bool)
                }
              }
              n225 = case shown="False" w122 {
                tunnel: w178 -> [w268 w269]
                tunnel: w136 -> [w267 _]
                tunnel: [w266 w269] -> w135
                frame False {
                  n226 = Insert Into Array(array=w268, new element=w267) -> (w266:dbl[][])  [unwired: 2 in]
                }
                frame True {
                }
              }
              "output array" <- w135
              n227 = Array Size(array=w135) -> (size(s)=w137:i32[])
              n228 = Index Array(array=w137) -> (element=w134:i32)  [unwired: 1 in]
              n229 = Greater Or Equal?(x=w134, y=200) -> (x >= y?=w142:bool)
              n230 = Equal?(x=w144, y=FALSE) -> (x = y?=w141:bool)
              n231 = Compound Arithmetic op=OR(w142, w141, w140) -> (w139:bool)
              "Time elapsed" <- w139
              n232 = Not(x=w139) -> (.not. x?=w138:bool)
              n233 = local write "Checkbox"(w138) -> ()
            }
          }
        }
      }
    }
    frame Error {
      (unwired) dbl[] [] ("DATA ARRAY")
    }
  }
  "DATA ARRAY OUT" <- w1
